vi "Fault_Logging.vi"(0 "String":string, 5 "Fault Table String Out":string[][](array[string]), 11 "error in (no error)":errorcluster) -> (15 "error out":errorcluster)   [LabVIEW 2016]
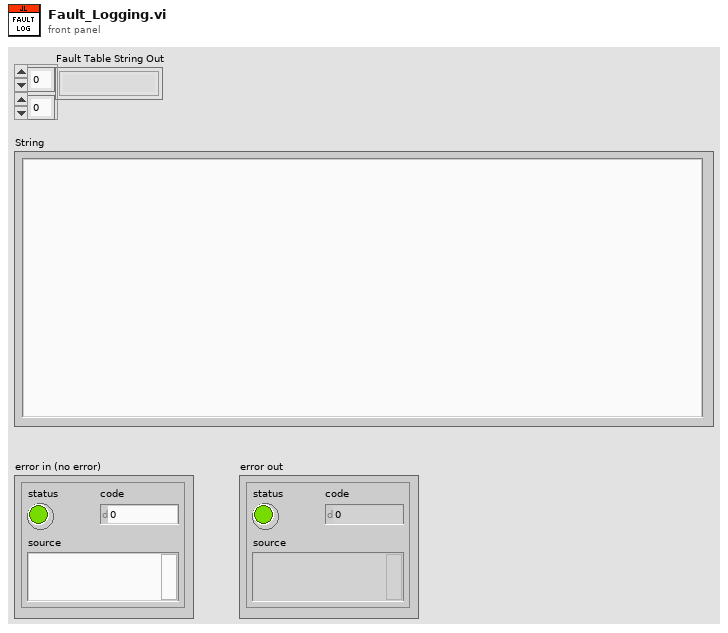
[diagram p1: front panel]
types:
  T1 = enum16{"open", "replace", "create", "open or create", "replace or create", "replace or create with confirmation"}
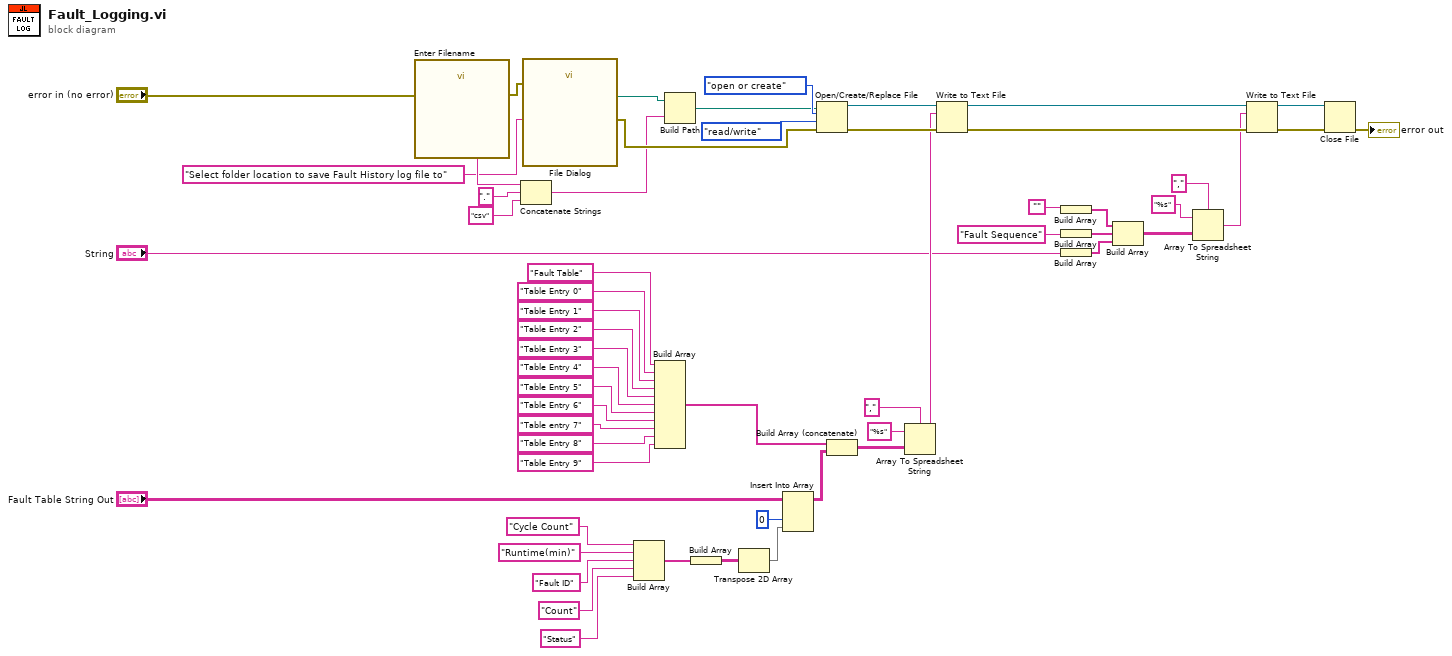
[diagram p0: block diagram]
diagram:
  n1 = call "Enter Filename"("error in (no error)"="error in (no error)") -> ("Filename"=w54:string, "error out"=w49:errorcluster)  [unwired: 16 in, 1 out]
  n2 = Concatenate Strings(w54, "." ("string"), "csv" ("string")) -> (w53:string)
  n3 = call "File Dialog"("prompt"="Select folder location to save Fault History log file to", "error in"=w49) -> ("selected path"=w34:path, "error out"=w55:errorcluster)  [unwired: 10 in, 2 out]
  n4 = Build Array("Cycle Count" ("delimiter (\\t)"), "Runtime(min)" ("delimiter (\\t)"), "Fault ID" ("delimiter (\\t)"), "Count" ("delimiter (\\t)"), "Status" ("delimiter (\\t)")) -> (w20:string[])
  n5 = Build Array("Fault Table" ("element"), "Table Entry 0" ("delimiter (\\t)"), "Table Entry 1" ("delimiter (\\t)"), "Table Entry 2" ("delimiter (\\t)"), "Table Entry 3" ("delimiter (\\t)"), "Table Entry 4" ("delimiter (\\t)"), "Table Entry 5" ("delimiter (\\t)"), "Table Entry 6" ("delimiter (\\t)"), "Table entry 7" ("delimiter (\\t)"), "Table Entry 8" ("delimiter (\\t)"), "Table Entry 9" ("delimiter (\\t)")) -> (w29:string[])
  n6 = Build Path(base path=w34, name or relative path=w53) -> (appended path=w36:path)
  n7 = Build Array(w20) -> (w19:string[][])
  n8 = Transpose 2D Array(2D array=w19) -> (transposed array=w17:string[][])
  n9 = Insert Into Array(array="Fault Table String Out", index (col)=0 ("disabled index (col)"), new element=w17) -> (w15:string[][])  [unwired: 1 in]
  n10 = Open/Create/Replace File(file path (use dialog)=w36, error in=w55, operation (0:open)=T1."open or create", access (0:read/write)=enum16{"read/write", "read-only", "write-only"}."read/write") -> (refnum out=w33:refnum<file>, error out=w32:errorcluster)  [unwired: 2 in, 1 out]
  n11 = Build Array (concatenate)(w29, w15) -> (w28:string[][])
  n12 = Array To Spreadsheet String(delimiter (Tab)=",", array=w28, 3:"%s" ("format string")) -> (spreadsheet string=w27:string)
  n13 = Write to Text File(file (use dialog)=w33, text=w27, error in=w32) -> (refnum out=w14:refnum<file>, error out=w13:errorcluster)  [unwired: 1 in, 1 out]
  n14 = Build Array("") -> (w1:string[])
  n15 = Build Array("Fault Sequence" ("element")) -> (w8:string[])
  n16 = Build Array("String") -> (w7:string[])
  n17 = Build Array(w1, w8, w7) -> (w6:string[][])
  n18 = Array To Spreadsheet String(delimiter (Tab)=",", array=w6, 3:"%s" ("format string")) -> (spreadsheet string=w3:string)
  n19 = Write to Text File(file (use dialog)=w14, text=w3, error in=w13) -> (refnum out=w11:refnum<file>, error out=w12:errorcluster)  [unwired: 1 in, 1 out]
  n20 = Close File(refnum=w11, error in=w12) -> (error out=→"error out":errorcluster)  [unwired: 1 out]
